vi "test from folder.vi"() -> ()   [LabVIEW 2018, in "Data Parser.lvclass"]
uses:
  Data Parser.lvclass
panel:
  out "valid":bool
  out "file index":i32
  out "file name":string
  out "same":bool
  out "frame string":string
  out "<f> string":string
  out "frame num":i32
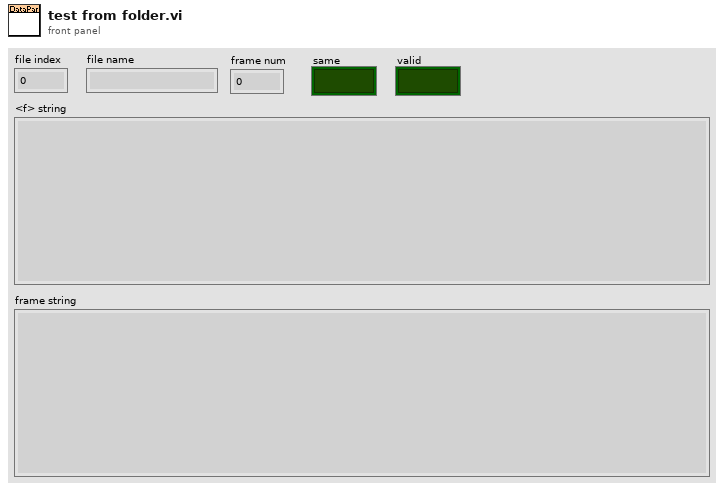
[diagram p1: front panel]
types:
  T1 = typedef "Data Parser.lvclass/frame data.ctl" = cluster{"Title":T2, "Basic Data":T3, "Sound":string, "<o> Data":T4, "<bp> Data":T5, "<c> Data":T6, "<w> Data":T7, "<i> Data Array":T8[], "<b> Data Array":T9[]}
  T2 = typedef "Data Parser.lvclass/frame title.ctl" = cluster{"Number":string, "Name":string}
  T3 = typedef "Data Parser.lvclass/frame basic data.ctl" = cluster{"Basic":cluster{"pic":string, "state":string, "wait":string, "next":string}, "Move":cluster{"dvx":string, "dvy":string, "dvz":string}, "Pic Center":cluster{"centerx":string, "centery":string}, "Skill":cluster{"hit_a":string, "hit_d":string, "hit_j":string, "hit_Fa":string, "hit_Ua":string, "hit_Da":string, "hit_Fj":string, "hit_Uj":string, "hit_Dj":string, "hit_ja":string}, "Mp":string}
  T4 = typedef "Data Parser.lvclass/frame o data.ctl" = cluster{"kind":string, "x":string, "y":string, "action":string, "dvx":string, "dvy":string, "dvz":string, "oid":string, "facing":string}
  T5 = typedef "Data Parser.lvclass/frame bp data.ctl" = cluster{"x":string, "y":string}
  T6 = typedef "Data Parser.lvclass/frame c data.ctl" = cluster{"kind":string, "x":string, "y":string, "injury":string, "cover":string, "vaction":string, "aaction":string, "taction":string, "hurtable":string, "decrease":string, "fronthurtact":string, "backhurtact":string, "dircontrol":string, "throwvx":string, "throwvy":string, "throwvz":string, "throwinjury":string}
  T7 = typedef "Data Parser.lvclass/frame w data.ctl" = cluster{"kind":string, "x":string, "y":string, "weaponact":string, "dvx":string, "dvy":string, "dvz":string, "attacking":string, "cover":string}
  T8 = typedef "Data Parser.lvclass/frame i data.ctl" = cluster{"kind":string, "x":string, "y":string, "w":string, "h":string, "dvx":string, "dvy":string, "dvz":string, "fall":string, "arest":string, "vrest":string, "bdefend":string, "injury":string, "zwidth":string, "effect":string, "catchingact":string, "caughtact":string}
  T9 = typedef "Data Parser.lvclass/frame b data.ctl" = cluster{"kind":string, "x":string, "y":string, "w":string, "h":string}
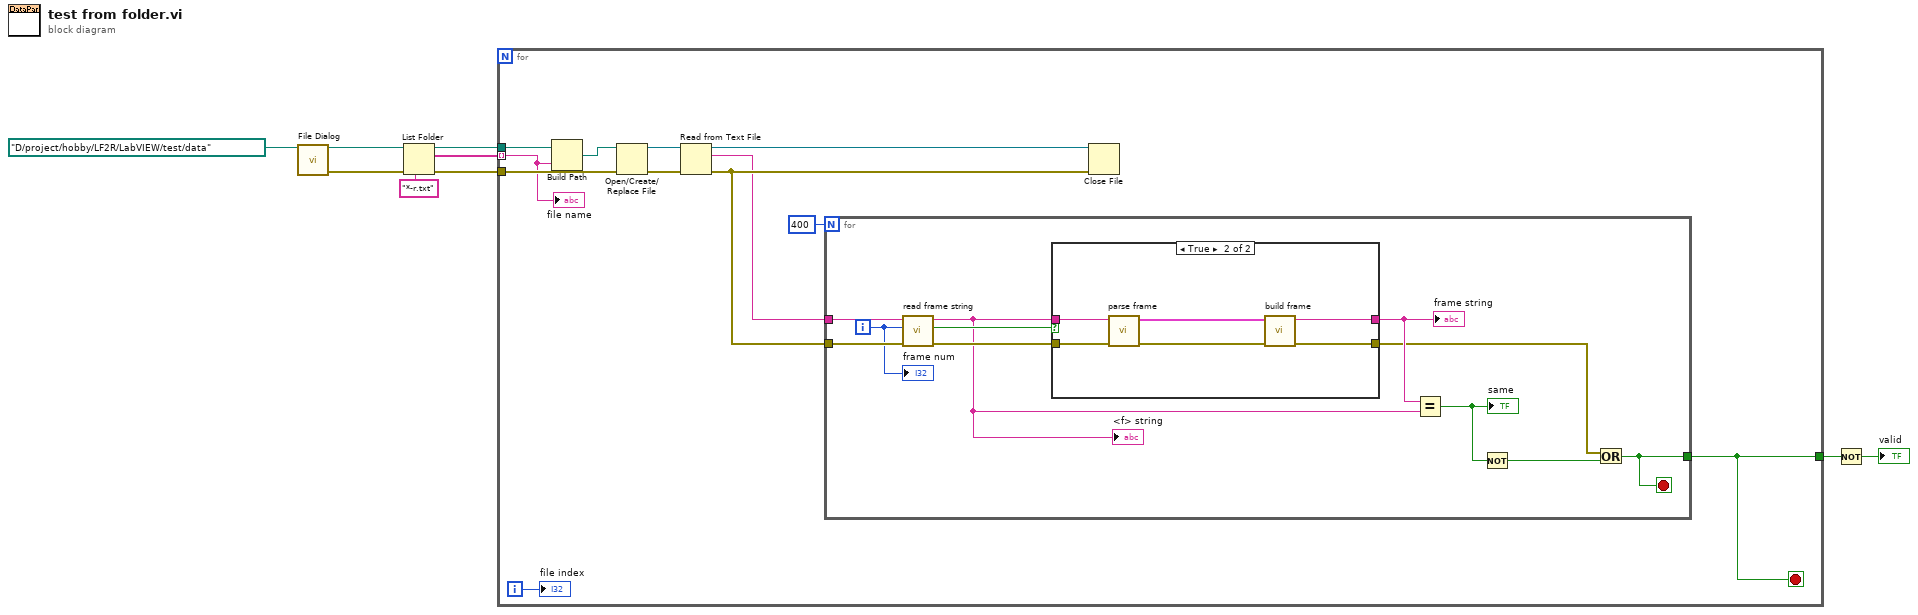
[diagram p0: block diagram]
diagram:
  n1 = call "File Dialog"("start path"=path "D:/project/hobby/LF2R/LabVIEW/test/data") -> ("selected path"=w8:path, "error out"=w6:errorcluster)  [unwired: 11 in, 2 out]
  n2 = List Folder(path=w8, pattern="*-r.txt" ("pattern (all files)"), error in=w6) -> (path out=w4:path, filenames=w3:string[], error out=w5:errorcluster)  [unwired: 1 in, 1 out]
  n3 = for {
    tunnel: w5 -> [w15]
    tunnel: w4 -> [w14]
    tunnel: w3 -> [w13] mode=indexing
    tunnel: [w10] -> w2
    i -> [w11]
    stop <- w10 stop-if-true
    n4 = Build Path(base path=w14, name or relative path=w13) -> (appended path=w12:path)
    n5 = Open/Create/Replace File(file path (use dialog)=w12, error in=w15) -> (refnum out=w21:refnum<file>, error out=w20:errorcluster)  [unwired: 4 in, 1 out]
    n6 = Read from Text File(file (use dialog)=w21, error in=w20) -> (refnum out=w19:refnum<file>, text=w17:string, error out=w18:errorcluster)  [unwired: 2 in, 1 out]
    n7 = for {
      N: 400 -> [_]
      tunnel: w18 -> [w31]
      tunnel: w17 -> [w30]
      tunnel: [w22] -> w10
      i -> [w29]
      stop <- w22 stop-if-true
      n8 = call "read frame string.vi"("error in"=w31, "frame number"=w29, "file string"=w30) -> ("error out"=w32:errorcluster, "found"=w28:bool, "<f> string"=w25:string)  [unwired: 5 in, 1 out]
      "<f> string" <- w25
      n9 = case shown="True" w28 {
        tunnel: w25 -> [w33 w38]
        tunnel: w32 -> [w34 w37]
        tunnel: [w33 w36] -> w27
        tunnel: [w34 w35] -> w26
        frame False {
        }
        frame True {
          n10 = call "parse frame.vi"("error in (no error)"=w37, "<f> string"=w38) -> ("error out"=w39:errorcluster, "frame data"=w40:T1)  [unwired: 8 in]
          n11 = call "build frame.vi"("error in (no error)"=w39, "frame data"=w40) -> ("error out"=w35:errorcluster, "<f> string"=w36:string)  [unwired: 8 in]
        }
      }
      "frame string" <- w27
      n12 = Equal?(x=w27, y=w25) -> (x = y?=w24:bool)
      "same" <- w24
      n13 = Not(x=w24) -> (.not. x?=w23:bool)
      n14 = Or(x=w26, y=w23) -> (x .or. y?=w22:bool)
      "frame num" <- w29
    }
    n15 = Close File(refnum=w19, error in=w18) -> ()  [unwired: 2 out]
    "file name" <- w13
    "file index" <- w11
  }
  n16 = Not(x=w2) -> (.not. x?=→"valid":bool)
